vi "test_WFCompose.vi"() -> ()   [LabVIEW 2009]
uses:
  random/impl/RandomArray_D.vi
panel:
  out "error out":errorcluster
  in  "Repetitions 4":T1
  in  "Repetitions 3":T1
  in  "Repetitions 2":T1
  in  "Repetitions 1":T1
  out "Rep4 Waveform Graph":waveform(dbl)(graph)
  out "Rep3 Waveform Graph":waveform(dbl)(graph)
  out "Rep2 Waveform Graph":waveform(dbl)(graph)
  out "Rep1 Waveform Graph":waveform(dbl)(graph)
  out "Waveform Out":waveform(dbl)
  out "Mother Waveform Graph":waveform(dbl)(graph)
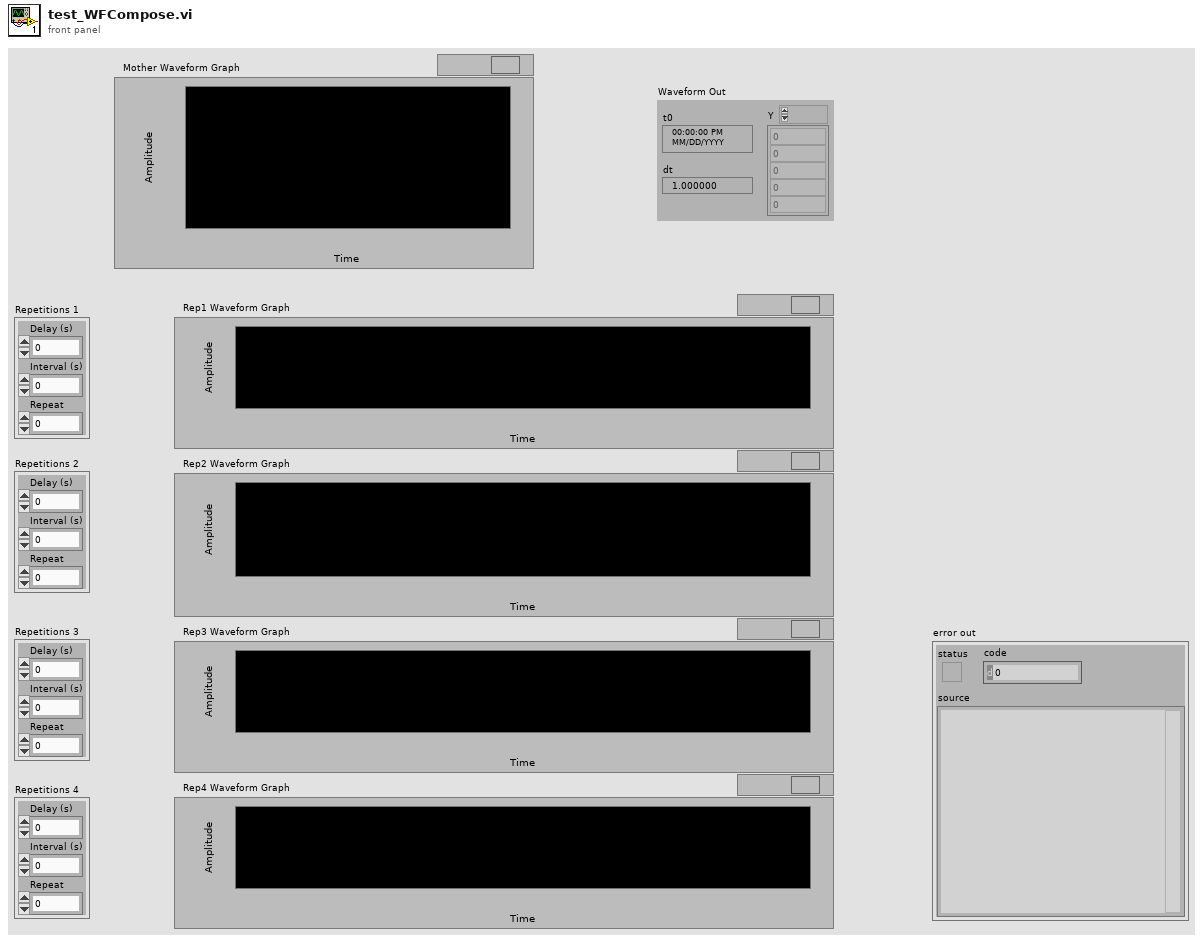
[diagram p1: front panel]
types:
  T1 = cluster{"Delay (s)":dbl, "Interval (s)":dbl, "Repeat":i32}
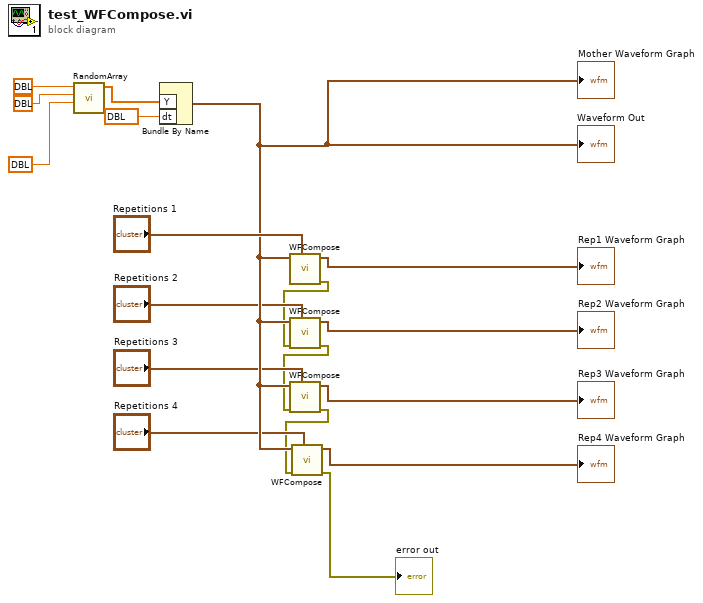
[diagram p0: block diagram]
diagram:
  n1 = call-poly "RandomArray.vi"("N"=dbl ?, "Min"=dbl ?, "Max 2"=dbl ? ("Max")) -> ("Array"=w9:dbl[])  [unwired: 8 in]
  n2 = Bundle By Name("Y"=w9, "dt"=dbl ?) -> (w8:waveform(dbl))  [unwired: 1 in]
  "Mother Waveform Graph" <- w8
  "Waveform Out" <- w8
  n3 = call "WFCompose.vi"("Repetitions"="Repetitions 1", "Waveform In"=w8) -> ("error out"=w4:errorcluster, "Analog Waveform Out"=→"Rep1 Waveform Graph":waveform(dbl))  [unwired: 8 in]
  n4 = call "WFCompose.vi"("Repetitions"="Repetitions 2", "error in (no error)"=w4, "Waveform In"=w8) -> ("error out"=w3:errorcluster, "Analog Waveform Out"=→"Rep2 Waveform Graph":waveform(dbl))  [unwired: 7 in]
  n5 = call "WFCompose.vi"("Repetitions"="Repetitions 3", "error in (no error)"=w3, "Waveform In"=w8) -> ("error out"=w2:errorcluster, "Analog Waveform Out"=→"Rep3 Waveform Graph":waveform(dbl))  [unwired: 7 in]
  n6 = call "WFCompose.vi"("Repetitions"="Repetitions 4", "error in (no error)"=w2, "Waveform In"=w8) -> ("error out"=→"error out":errorcluster, "Analog Waveform Out"=→"Rep4 Waveform Graph":waveform(dbl))  [unwired: 7 in]
